vi "SmartEdge.vi"(7 "init":bool, 9 "Filter Length":i32, 11 "in":bool) -> (3 "edge":bool)   [LabVIEW 2019, in "Stand.lvclass"]
uses:
  Stand.lvclass
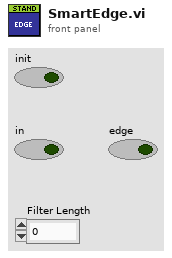
[diagram p1: front panel]
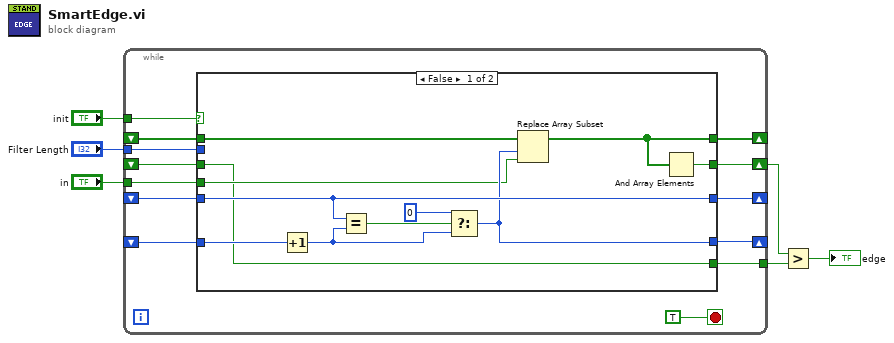
[diagram p0: block diagram]
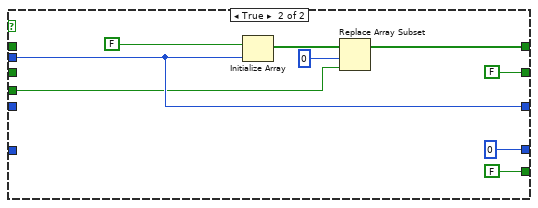
[diagram p2: hidden frame]
diagram:
  n1 = while {
    tunnel: "init" -> [w18]
    shift-right: [w16] -> _
    shift-left: _ -> [w11]
    tunnel: "Filter Length" -> [w17]
    shift-right: [w15] -> _
    shift-left: _ -> [w12]
    shift-right: [w14] -> _
    shift-left: _ -> [w13]
    tunnel: "in" -> [w10]
    shift-right: [w9] -> w5
    shift-left: _ -> [w8]
    tunnel: [w7] -> w1
    stop <- TRUE stop-if-true
    n2 = case shown="False" w18 {
      tunnel: w17 -> [_ w37]
      tunnel: [w22 w35] -> w16
      tunnel: [w28 w37] -> w15
      tunnel: [w24 0] -> w14
      tunnel: w13 -> [w30 _]
      tunnel: w12 -> [w28 _]
      tunnel: w11 -> [w25 _]
      tunnel: w10 -> [w23 w34]
      tunnel: [w21 FALSE] -> w9
      tunnel: w8 -> [w20 _]
      tunnel: [w20 FALSE] -> w7
      frame False {
        n3 = Increment(x=w30) -> (x+1=w27:i32)
        n4 = Equal?(x=w28, y=w27) -> (x = y?=w29:bool)
        n5 = Select(t=0, s=w29, f=w27) -> (s? t:f=w24:i32)
        n6 = Replace Array Subset(array=w25, new element=w23, index=w24) -> (w22:bool[])
        n7 = And Array Elements(Boolean array=w22) -> (logical AND=w21:bool)
      }
      frame True {
        n8 = Initialize Array(FALSE, w37) -> (w39:bool[])
        n9 = Replace Array Subset(array=w39, new element=w34, index=0) -> (w35:bool[])
      }
    }
  }
  n10 = Greater?(x=w5, y=w1) -> (0:→"edge":bool)
